vi "stop_and_free_dmd.vi"(11 "DevId":u32) -> (3 "return array2":i32[](array[numeric]))   [LabVIEW 2019]
uses:
  <userlib>/alp4395/alp4395.lvlib
panel:
  out "function return 11":i32
  out "function return 10":i32
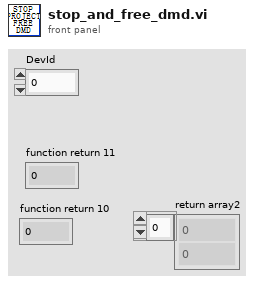
[diagram p1: front panel]
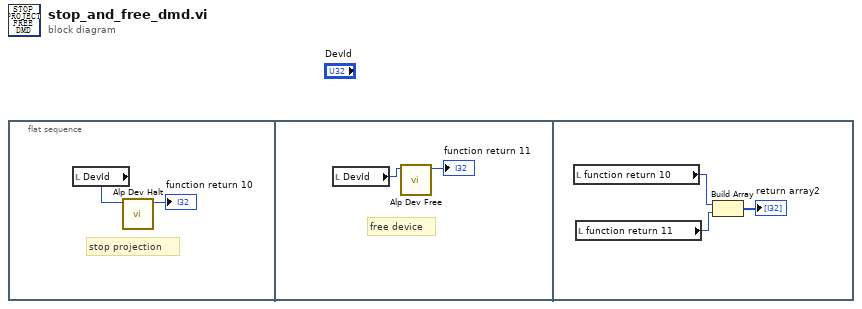
[diagram p0: block diagram]
diagram:
  n1 = flat-sequence {
    frame #0 {
      # "stop projection"
      n2 = local read "DevId"() -> (w2:u32)
      n3 = call <userlib>:"Alp Dev Halt.vi"("DeviceId"=w2) -> ("function return"=→"function return 10":i32)  [unwired: 9 in, 1 out]
    }
    frame #1 {
      # "free device"
      n4 = local read "DevId"() -> (w4:u32)
      n5 = call <userlib>:"Alp Dev Free.vi"("DeviceId"=w4) -> ("function return"=→"function return 11":i32)  [unwired: 9 in, 1 out]
    }
    frame #2 {
      n6 = local read "function return 10"() -> (w5:i32)
      n7 = local read "function return 11"() -> (w6:i32)
      n8 = Build Array(w5, w6) -> (→"return array2":i32[])
    }
  }
